vi "Reset All Valves.vi"   [LabVIEW 2015]
uses:
  Valve Button Mapping Global Action.ctl
types:
  T1 = typedef "Valve Button Mapping Global Action.ctl" = enum16{"Get", "Set", "Init", "Reset All", "Reset to Standby"}
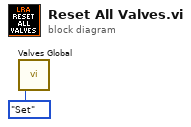
[diagram p0: block diagram]
diagram:
  n1 = call "Valves Global.vi"("Action"=Valve_Button_Mapping_Global_Action."Set") -> ()  [unwired: 7 in, 4 out]
